vi "PDash - Add New DQMH Module.vi"(4 "New Module Name":string, 6 "New Module Folder":path, 9 "External Module Info":T1, 10 "New Module Type":T3, 11 "Project":refnum<vi>) -> (0 "error out":errorcluster)   [LabVIEW 2020]
doc: "_____\nCreated using DQMH Event Scripter 7.1.0.1447."
uses:
  <vilib>/Delacor/Delacor QMH/Libraries/_Scripting Support/Module Type (Including External)--enum.ctl
  <vilib>/Delacor/Delacor QMH/Libraries/_Scripting Support/External Module Info--cluster.ctl
  <vilib>/Delacor/Delacor QMH/Libraries/_Scripting Support/Module Type--enum.ctl
  PantherDashboard Scripting Hooks/Panther Dasboard Scripting Hooks.lvlib
  <vilib>/Delacor/Delacor QMH/Libraries/_Scripting Support/dqmh_lib_DQMH Scripting Support.lvlib
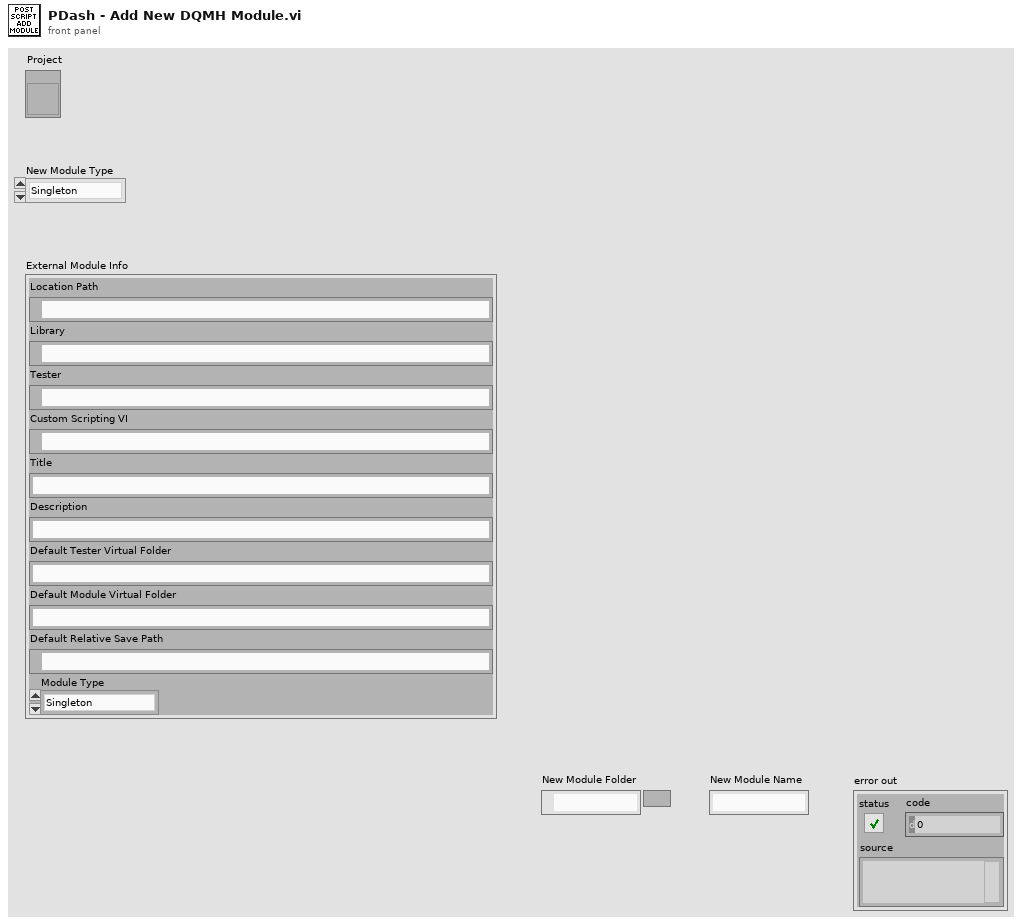
[diagram p1: front panel]
types:
  T1 = typedef "dqmh_lib_DQMH Scripting Support.lvlib/External Module Info--cluster.ctl" = cluster{"Location Path":path, "Library":path, "Tester":path, "Custom Scripting VI":path, "Title":string, "Description":string, "Default Tester Virtual Folder":string, "Default Module Virtual Folder":string, "Default Relative Save Path":path, "Module Type":T2}
  T2 = typedef "dqmh_lib_DQMH Scripting Support.lvlib/Module Type--enum.ctl" = enum16{"Singleton", "Cloneable"}
  T3 = typedef "dqmh_lib_DQMH Scripting Support.lvlib/Module Type (Including External)--enum.ctl" = enum16{"Singleton", "Cloneable", "External"}
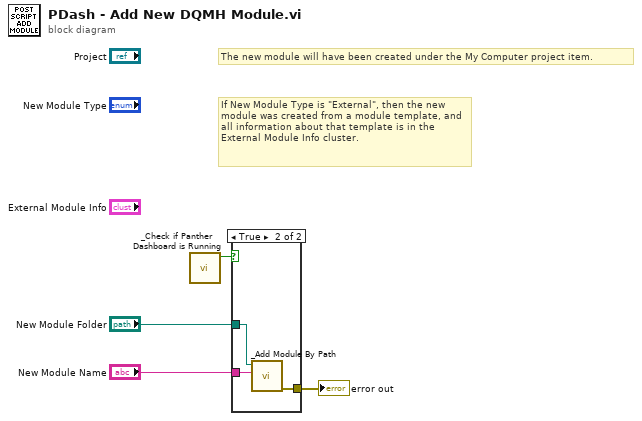
[diagram p0: block diagram]
diagram:
  # "If New Module Type is \"External\", then the new module was created from a module template, and all information about that template is in the External Module Info cluster."
  # "The new module will have been created under the My Computer project item."
  n1 = call "_Check if Panther Dashboard is Running.vi"() -> ("Panther Dashboard is Running?"=w1:bool)  [unwired: 10 in, 1 out]
  n2 = case shown="True" w1 {
    tunnel: [_ w7] -> w4
    tunnel: "New Module Folder" -> [_ w5]
    tunnel: "New Module Name" -> [_ w6]
    frame False {
    }
    frame True {
      n3 = call "_Add Module By Path.vi"("New Module Name"=w6, "New Module Folder"=w5) -> ("error out"=w7:errorcluster)  [unwired: 9 in]
    }
  }
  "error out" <- w4
